vi "Read_PDU_SOFT.vi"(8 "errin":errorcluster, 11 "ECU number":u32=1) -> (0 "error out":errorcluster, 3 "SN":string)   [LabVIEW 2020]
uses:
  C/Program Files (x86)/National Instruments/LabVIEW 2020/user.lib/PCAN Basic/Controls/BaudrateEenum.ctl
  C/Program Files (x86)/National Instruments/LabVIEW 2020/user.lib/PCAN Basic/Controls/Channel.ctl
  C/Program Files (x86)/National Instruments/LabVIEW 2020/user.lib/PCAN Basic/PCANBasic.lvlib
panel:
  out "MDP OK":bool
  out "IDOK":bool
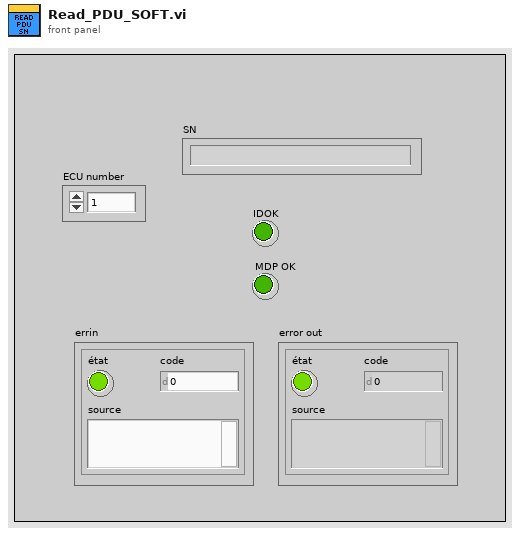
[diagram p1: front panel]
types:
  T1 = typedef "PCANBasic.lvlib/Channel.ctl" = enum16{"PCAN_NONEBUS", "not used1", "not used2", "not used3", "not used4", "not used5", "not used6", "not used7", "not used8", "not used9", "not used10", "not used11", "not used12", "not used13", "not used14", "not used15", "not used16", "not used17", "not used18", "not used19", "not used20", "not used21", "not used22", "not used23", "not used24", "not used25", "not used26", "not used27", "not used28", "not used29", "not used30", "not used31", "not used32", "PCAN_ISABUS1", "PCAN_ISABUS2", "PCAN_ISABUS3", "PCAN_ISABUS4", "PCAN_ISABUS5", "PCAN_ISABUS6", "PCAN_ISABUS7", "PCAN_ISABUS8", "not used41", "not used42", "not used43", "not used44", "not used45", "not used46", "not used47", "not used48", "PCAN_DNGBUS1", "not used50", "not used51", "not used52", "not used53", "not used54", "not used55", "not used56", "not used57", "not used58", "not used59", "not used60", "not used61", "not used62", "not used63", "not used64", "PCAN_PCIBUS1", "PCAN_PCIBUS2", "PCAN_PCIBUS3", "PCAN_PCIBUS4", "PCAN_PCIBUS5", "PCAN_PCIBUS6", "PCAN_PCIBUS7", "PCAN_PCIBUS8", "not used73", "not used74", "not used75", "not used76", "not used77", "not used78", "not used79", "not used80", "PCAN_USBBUS1", "PCAN_USBBUS2", "PCAN_USBBUS3", "PCAN_USBBUS4", "PCAN_USBBUS5", "PCAN_USBBUS6", "PCAN_USBBUS7", "PCAN_USBBUS8", "Not used89", "Not used90", "Not used91", "Not used92", "Not used93", "Not used94", "Not used95", "Not used96", "PCAN_PCCBUS1", "PCAN_PCCBUS2"}
  T2 = typedef "PCANBasic.lvlib/BaudrateEenum.ctl" = enum16{"CAN_Baud_1M", "CAN_Baud_800K", "CAN_BAUD_500K", "CAN_BAUD_250K", "CAN_BAUD_125K", "CAN_BAUD_100K", "CAN_BAUD_95K", "CAN_BAUD_83K", "CAN_BAUD_50K", "CAN_BAUD_47K", "CAN_BAUD_33K", "CAN_BAUD_20K", "CAN_BAUD_10K", "CAN_BAUD_5K", "User Baudrate"}
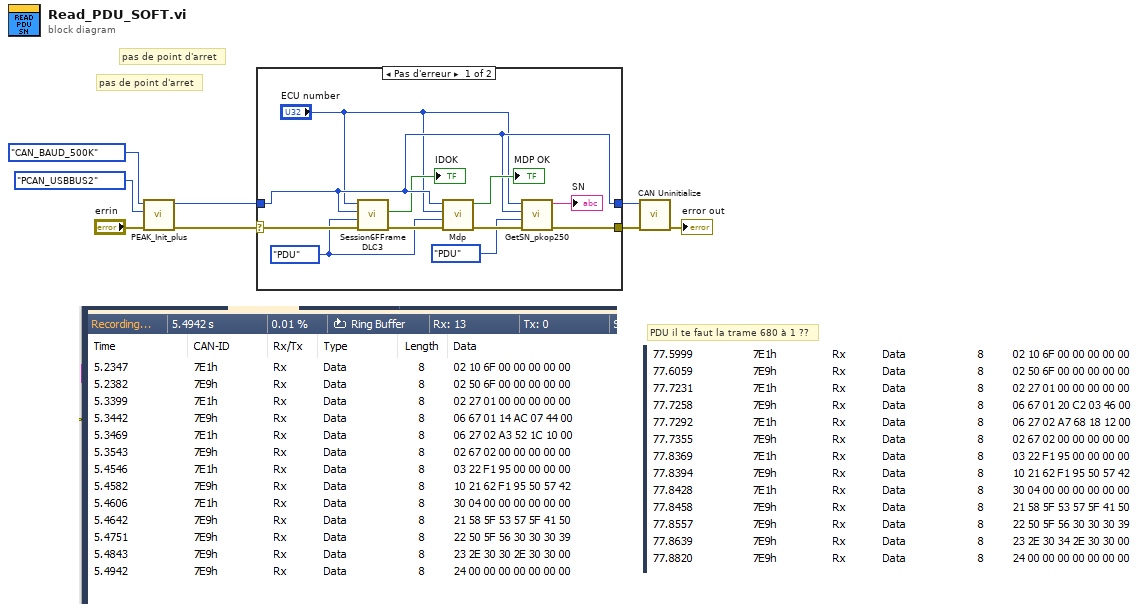
[diagram p0: block diagram]
diagram:
  # "pas de point d'arret"
  # "pas de point d'arret"
  # "PDU il te faut la trame 680 à 1 ??"
  n1 = call "PEAK_Init_plus.vi"("errin"="errin", "Channel"=Channel."PCAN_USBBUS2", "BTR0BTR1"=BaudrateEenum."CAN_BAUD_500K") -> ("errout"=w3:errorcluster, "Channel out"=w2:T1)  [unwired: 7 in]
  n2 = case shown="Pas d'erreur" w3 {
    selector: w3 -> [w15 w21]
    tunnel: [w17 w21] -> w7
    tunnel: w2 -> [w14 w20]
    tunnel: [w14 w20] -> w1
    frame No Error {
      w10 = enum16{"PDU", "CMOD"}."PDU" ("Énum")
      n3 = call "Session6FFrameDLC3.vi"("errin"=w15, "Énum"=w10, "ChanelIn"=w14, "IDnumber"="ECU number") -> ("errout"=w13:errorcluster, "Identique"=→"IDOK":bool)  [unwired: 4 in, 2 out]
      n4 = call "Mdp.vi"("errin"=w13, "Énum"=w10, "CMODNum"="ECU number", "Channel out"=w14) -> ("errout"=w18:errorcluster, "OK"=→"MDP OK":bool)  [unwired: 6 in]
      n5 = call "GetSN_pkop250.vi"("err in"=w18, "TypeCible"=enum16{"CMOD", "BMS", "PDU"}."PDU", "Channel in"=w14, "ECU Numb"="ECU number") -> ("errout"=w17:errorcluster, "Chaîne"=→"SN":string)  [unwired: 6 in]
    }
    frame Error {
    }
  }
  n6 = call "CAN Uninitialize.vi"("error in (no error)"=w7, "Channel"=w1) -> ("error out"=→"error out":errorcluster)  [unwired: 7 in, 2 out]
